vi "test1.vi"(11 "Cluster":T1 {"frequency shift" format="%#_30g"}) -> (3 "output cluster":T1 {"frequency shift" format="%#_30g"})   [LabVIEW 2021]
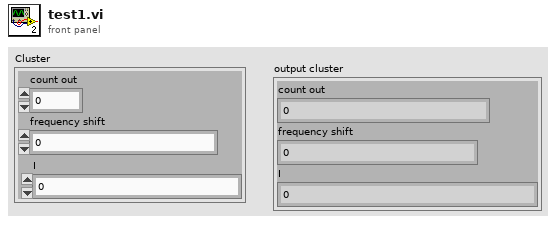
[diagram p1: front panel]
types:
  T1 = cluster{"count out":u32, "frequency shift":fxp<+/-,48,0>, "I":fxp<+/-,18,1>}
  T2 = cluster{u32, "frequency shift":fxp<+/-,48,0>, "I":fxp<+/-,18,1>}
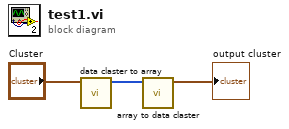
[diagram p0: block diagram]
diagram:
  n1 = call "data claster to array.vi"("Cluster"="Cluster") -> ("Array"=w2:u64[])  [unwired: 10 in]
  n2 = call "array to data claster.vi"("Array"=w2) -> ("Cluster"=→"output cluster":T2)  [unwired: 10 in]
